vi "PythonNode_CHR2.vi"() -> ()   [LabVIEW 2022 SP3]
doc: "This example demonstrates how to call a Python function and pass arguments as numpy arrays. It uses a python function to compute the product of two matrices."
uses:
  support/PythonVersionsEnum.ctl
  <vilib>/Utility/file.llb/Read Delimited Spreadsheet (DBL).vi
panel:
  out "Likely CHR2 response?":bool
  out "Likely CHR2 induced response?":dbl
  out "Time to peak from stimulus onset\n(ms)":dbl
  out "Abs. Spike Amplitude\n(mV)":dbl
  out "Peak spike magnitude\n(mv)":dbl
  out "Peak amp.      Spike amp.    Time to Peak":dbl[](array[numeric])
  out "time_ms":dbl[](array[numeric])
  out "digital_V":dbl[](array[numeric])
  out "voltage_mV":dbl[](array[numeric])
  in  "path to python module":path
  out "return value 4":dbl[](array[numeric])
  out "return value 3":dbl[](array[numeric])
  out "return value":dbl[](array[numeric])
  out "Waveform Graph":dbl[][](graph)
  out "all rows":dbl[][](array[numeric])
  in  "file path to analysis file":path
  out "python error out":errorcluster
  in  "python error in (no error)":errorcluster
  in  "python version":T1
  # "Overview: Demonstrates how to call a Python function and pass arrays as numpy arrays.\nRequirements: Python 3.6, 3.7, 3.8 or 3.9 with the same bitness as LabVIEW with numpy installed.\nInstructions:\n1. Set the Python version to the version of Python you want to execute code in.\n2. Run the VI. You should see the result of multiplying the matrix  \"a\" by the matrix \"b\" in the indicator \"a*b\".\n3. See comments on the block diagram of this VI and in \"ExamplePythonModule.py\" for more information about how the call python node passes arguments and handles return values."
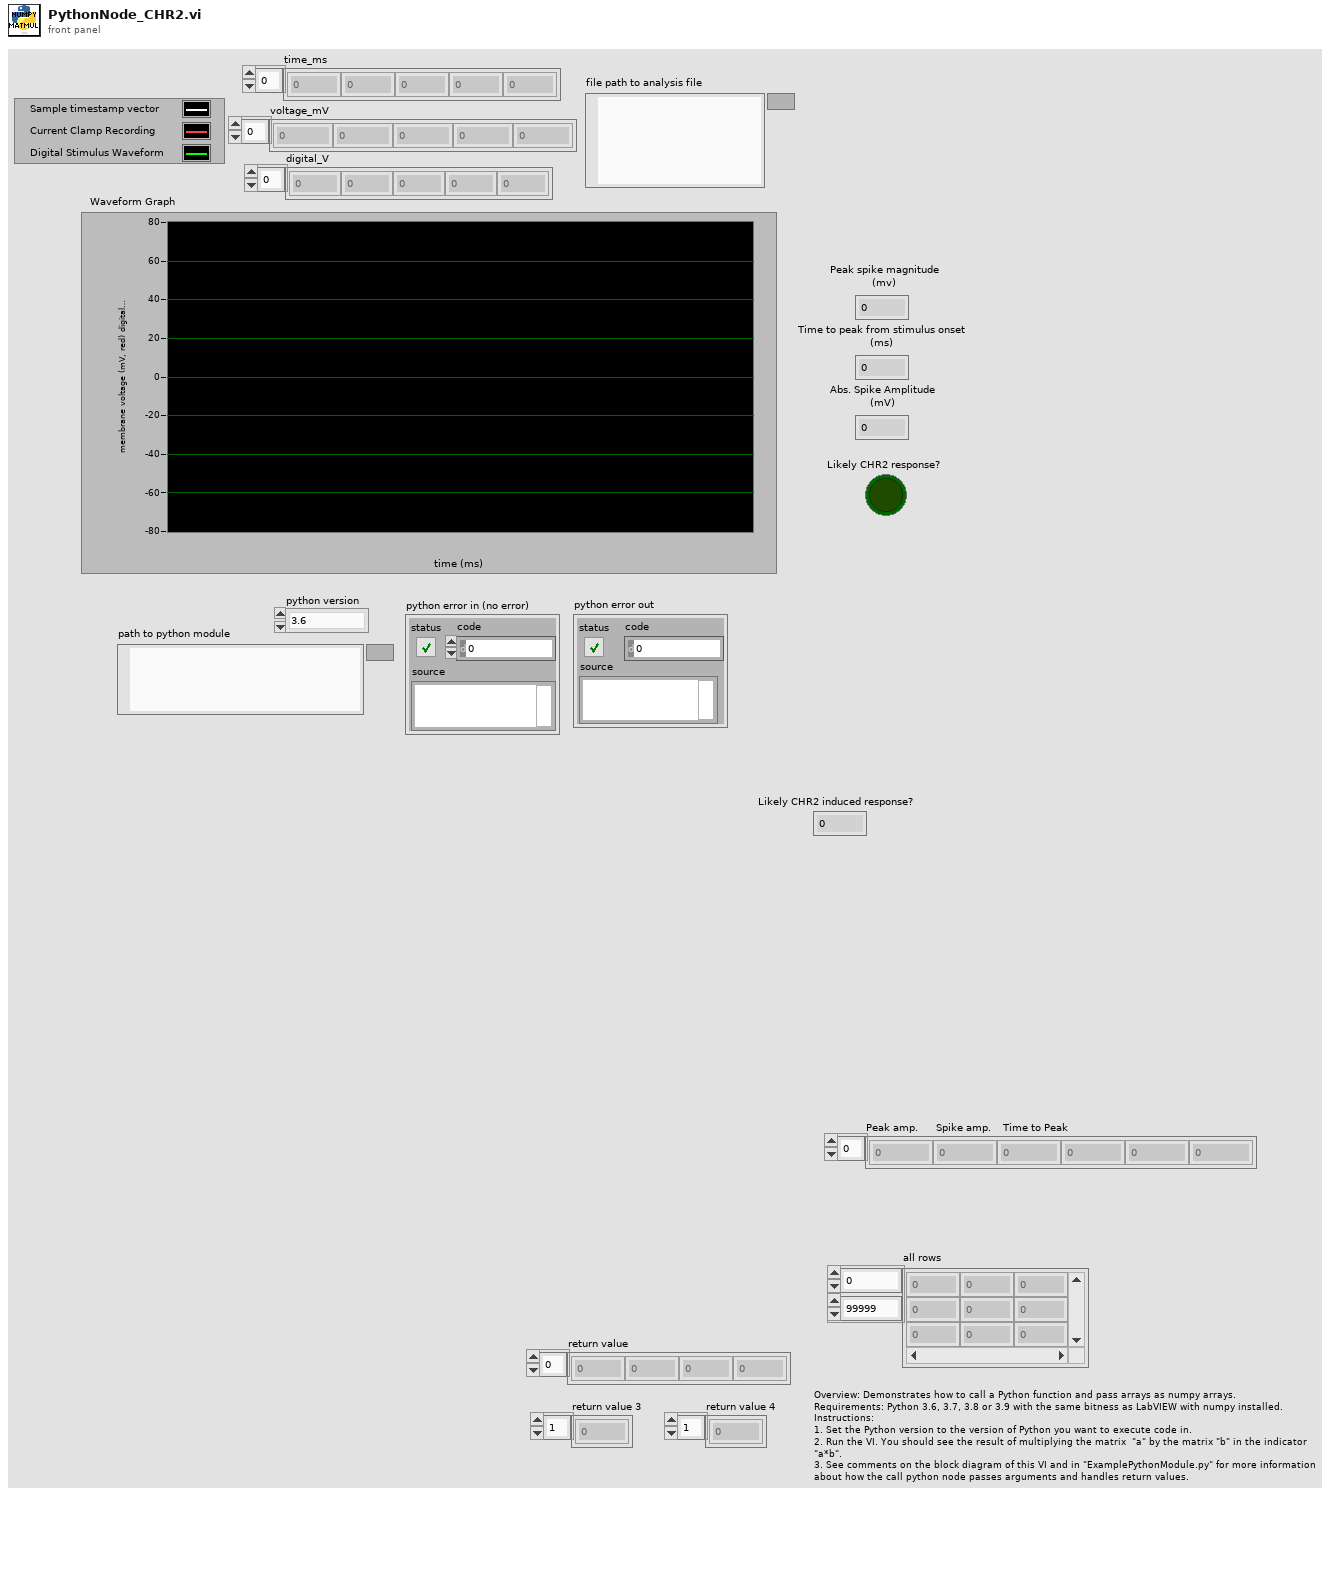
[diagram p1: front panel]
types:
  T1 = typedef "PythonVersionsEnum.ctl" = enum16{"3.6", "3.7", "3.8", "3.9"}
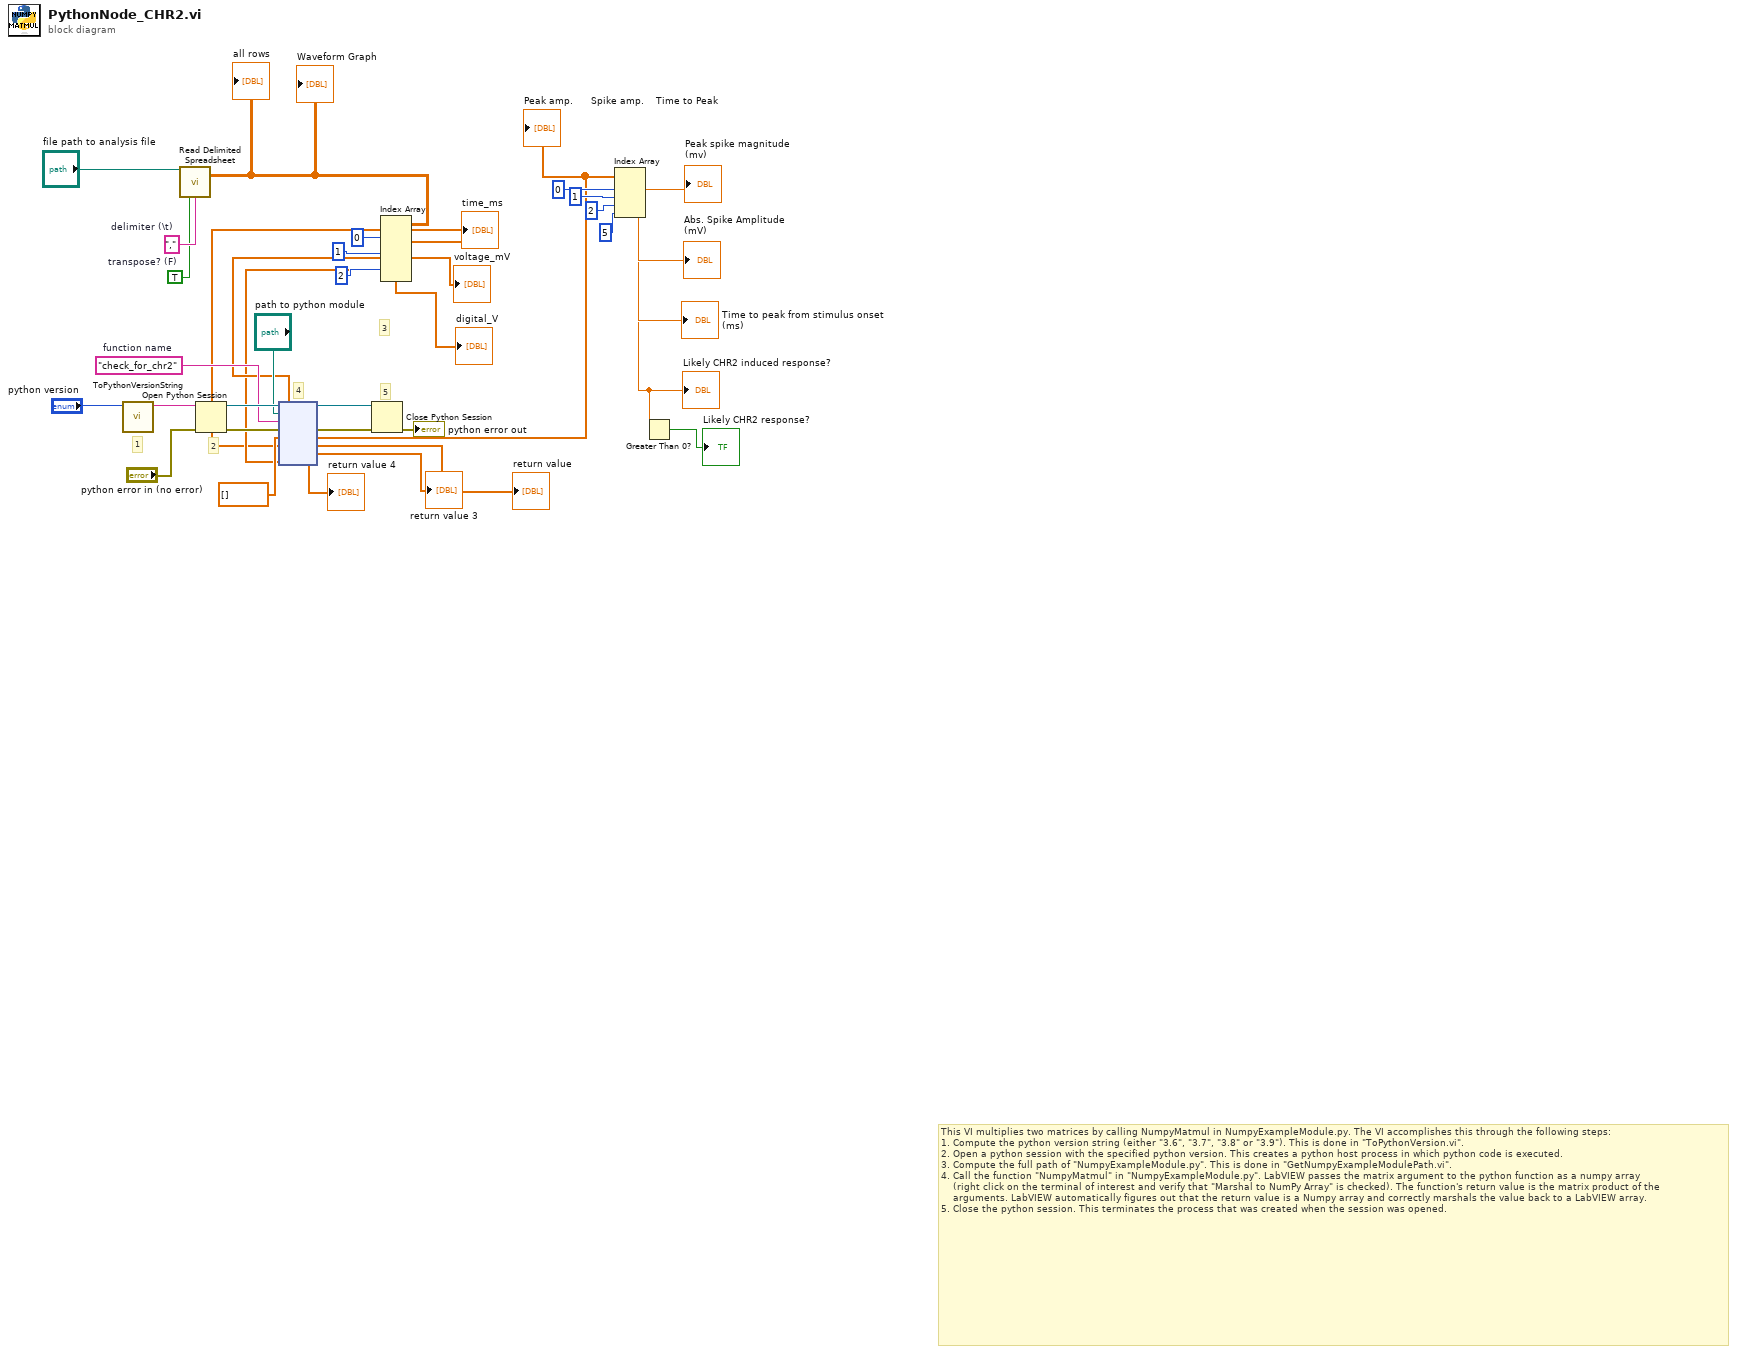
[diagram p0: block diagram]
diagram:
  w23 = TRUE  # transpose? (F)
  w24 = ","  # delimiter (\t)
  w29 = "check_for_chr2"  # function name
  # "5"
  # "4"
  # "2"
  # "3"
  # "1"
  # "This VI multiplies two matrices by calling NumpyMatmul in NumpyExampleModule.py. The VI accomplishes this through the following steps:\n1. Compute the python version string (either \"3.6\", \"3.7\", \"3.8\" or \"3.9\"). This is done in \"ToPythonVersion.vi\". \n2. Open a python session with the specified python version. This creates a python host process in which python code is executed.\n3. Compute the full path of \"NumpyExampleModule.py\". This is done in \"GetNumpyExampleModulePath.vi\".\n4. Call the function \"NumpyMatmul\" in \"NumpyExampleModule.py\". LabVIEW passes the matrix argument to the python function as a numpy array\n    (right click on the terminal of interest and verify that \"Marshal to NumPy Array\" is checked). The function's return value is the matrix product of the\n    arguments. LabVIEW automatically figures out that the return value is a Numpy array and correctly marshals the value back to a LabVIEW array.\n5. Close the python session. This terminates the process that was created when the session was opened."
  n1 = call "ToPythonVersionString.vi"("python version"="python version") -> ("python version string"=w34:string)  [unwired: 10 in]
  n2 = call-poly <vilib>:"Read Delimited Spreadsheet.vi"("file path (dialog if empty)"="file path to analysis file", "transpose? (F)"=w23, "delimiter (\\t)"=w24) -> ("all rows"=w19:dbl[][])  [unwired: 7 in, 5 out]
  "all rows" <- w19
  "Waveform Graph" <- w19
  n3 = Open Python Session(python version=w34, 3:"python error in (no error)") -> (session out=w31:refnum<k35>, error out=w30:errorcluster)  [unwired: 1 in]
  n4 = Index Array(array=w19, index (row) #1=0 ("index"), index (row) #2=1 ("index"), index (row) #3=2 ("index")) -> (element #1=w1:dbl[], element #2=w15:dbl[], element #3=w2:dbl[])  [unwired: 3 in]
  "voltage_mV" <- w15
  "digital_V" <- w2
  "time_ms" <- w1
  n5 = node(w31, "path to python module", w29, w30, dbl[] [] ("b"), w1, w15, w2) -> (w28:refnum<k35>, w27:errorcluster, w5:dbl[], →"return value":dbl[], →"return value 3":dbl[], →"return value 4":dbl[])  [unwired: 2 out]
  "Peak amp.      Spike amp.    Time to Peak" <- w5
  n6 = Close Python Session(session in=w28, error in=w27) -> (11:→"python error out":errorcluster)
  n7 = Index Array(array=w5, index #1=0, index #2=1, index #3=2, index #4=5) -> (element #1=→"Peak spike magnitude\n(mv)":dbl, element #2=→"Abs. Spike Amplitude\n(mV)":dbl, element #3=→"Time to peak from stimulus onset\n(ms)":dbl, element #4=w3:dbl)
  "Likely CHR2 induced response?" <- w3
  n8 = Greater Than 0?(x=w3) -> (x > 0?=→"Likely CHR2 response?":bool)
